vi "Create Digraph String.vi"(8 "Show Tag Labels?":bool, 9 "tag info":T3(array[cluster]), 10 "tables html":string[](array[string]), 11 "channel and node pairs":T1[](array[typedef])) -> (3 "digraph output":string)   [LabVIEW 2014, in "GraphViz Mapping Visualizer.lvlib"]
uses:
  GraphViz Mapping Visualizer.lvlib
  <vilib>/NI/Tag Bus/tag/Data Type.ctl
  Channel to Port Pair.ctl
  <vilib>/NI/Tag Bus/tag/tag descriptor.lvclass
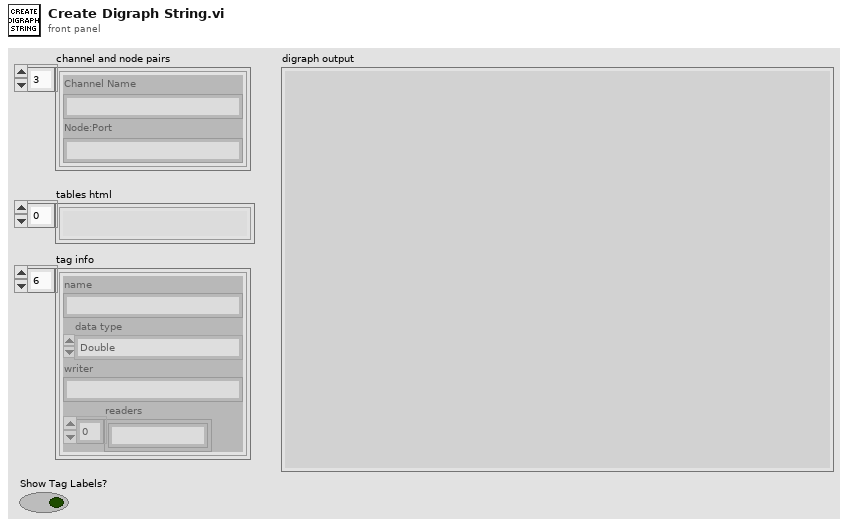
[diagram p1: front panel]
types:
  T1 = typedef "GraphViz Mapping Visualizer.lvlib/Channel to Port Pair.ctl" = cluster{"Channel Name":string, "Node:Port":string}
  T2 = typedef "tag bus.lvlib/tag descriptor.lvclass/Data Type.ctl" = enum16{"Double", "Single", "I64", "I32", "I16", "I8", "U64", "U32", "U16", "U8", "Boolean", "String", "Array of Double", "Array of Single", "Array of I64", "Array of I32", "Array of I16", "Array of I8", "Array of U64", "Array of U32", "Array of U16", "Array of U8", "Array of Boolean", "Array of String"}
  T3 = cluster{"name":string, "data type":T2, "writer":string, "readers":string[]}[]
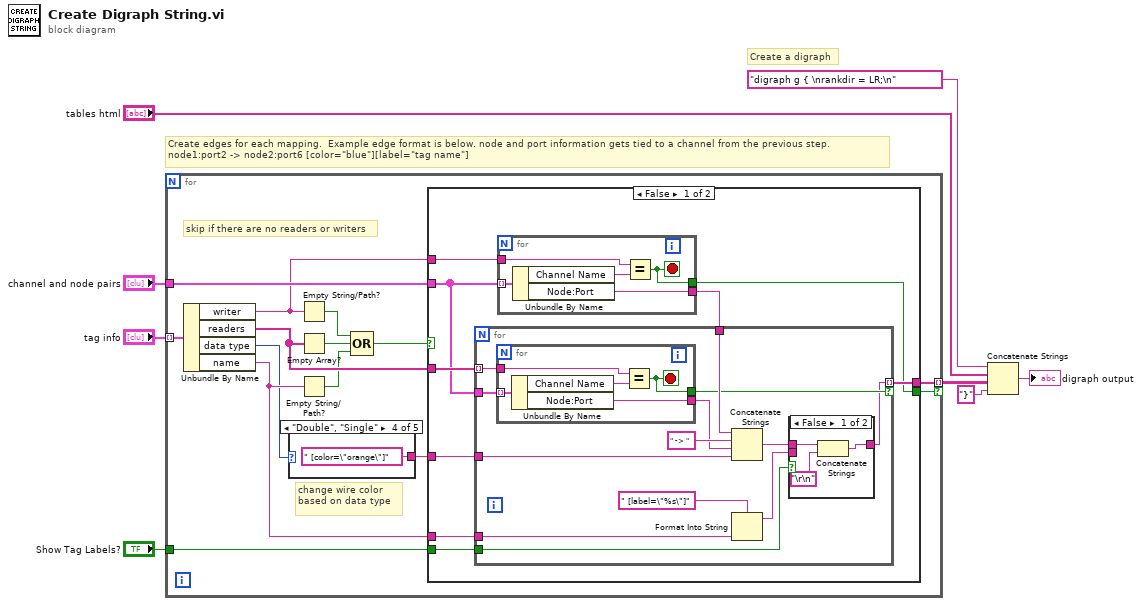
[diagram p0: block diagram]
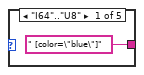
[diagram p2: hidden frame]
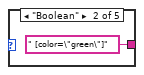
[diagram p3: hidden frame]
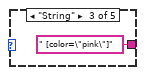
[diagram p4: hidden frame]
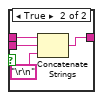
[diagram p6: hidden frame]
diagram:
  # "Create a digraph"
  # "Create edges for each mapping.  Example edge format is below. node and port information gets tied to a channel from the previous step.\nnode1:port2 -> node2:port6 [color=\"blue\"][label=\"tag name\"]"
  n1 = for {
    tunnel: "channel and node pairs" -> [w20]
    tunnel: [w19] -> w6 mode=indexing if=w18
    tunnel: "Show Tag Labels?" -> [w17]
    tunnel: "tag info" -> [w16] mode=indexing
    # "change wire color based on data type"
    # "skip if there are no readers or writers"
    n2 = Unbundle By Name(w16) -> ("writer"=w15:string, "readers"=w14:string[], "data type"=w9:T2, "name"=w12:string)
    n3 = case shown="\"Double\", \"Single\"" w9 {
      tunnel: [" [color=\"blue\"]" ("string") " [color=\"green\"]" ("string") " [color=\"pink\"]" ("string") " [color=\"orange\"]" ("string") _] -> w10
      frame "I64".."U8" {
      }
      frame "Boolean" {
      }
      frame "String" {
      }
      frame "Double", "Single" {
      }
      frame Default {
      }
    }
    n4 = Empty String/Path?(string/path=w15) -> (empty?=w13:bool)
    n5 = Empty Array?(array=w14) -> (empty?=w22:bool)
    n6 = Empty String/Path?(string/path=w12) -> (empty?=w11:bool)
    n7 = Compound Arithmetic op=OR(w13, w22, w11) -> (w21:bool)
    n8 = case shown="False" w21 {
      tunnel: w20 -> [w34 _]
      tunnel: w14 -> [w35 _]
      tunnel: w15 -> [w33 _]
      tunnel: w12 -> [w31 _]
      tunnel: [w30 _] -> w19
      tunnel: [w29 _] -> w18
      tunnel: w17 -> [w28 _]
      tunnel: w10 -> [w27 _]
      frame False {
        n9 = for {
          tunnel: w33 -> [w38]
          tunnel: w34 -> [w40] mode=indexing
          tunnel: [w37] -> w29
          tunnel: [w36] -> w32
          stop <- w37 stop-if-true
          n10 = Unbundle By Name(w40) -> ("Channel Name"=w39:string, "Node:Port"=w36:string)
          n11 = Equal?(x=w38, y=w39) -> (x = y?=w37:bool)
        }
        n12 = for {
          tunnel: w35 -> [w53] mode=indexing
          tunnel: w34 -> [w52]
          tunnel: w32 -> [w51]
          tunnel: w31 -> [w48]
          tunnel: [w42] -> w30 mode=indexing if=w46
          tunnel: w28 -> [w45]
          tunnel: w27 -> [w41]
          n13 = for {
            tunnel: w53 -> [w63]
            tunnel: w52 -> [w65] mode=indexing
            tunnel: [w62] -> w46
            tunnel: [w61] -> w47
            stop <- w62 stop-if-true
            n14 = Unbundle By Name(w65) -> ("Channel Name"=w64:string, "Node:Port"=w61:string)
            n15 = Equal?(x=w63, y=w64) -> (x = y?=w62:bool)
          }
          n16 = Concatenate Strings(w51, " -> " ("string"), w47, w41) -> (w43:string)
          n17 = Format Into String(format string=" [label=\"%s\"]" ("string"), w48) -> (resulting string=w44:string)  [unwired: 2 in, 1 out]
          n18 = case shown="False" w45 {
            tunnel: w44 -> [_ w59]
            tunnel: w43 -> [w56 w60]
            tunnel: [w54 w58] -> w42
            frame False {
              n19 = Concatenate Strings(w56, "\r\n") -> (w54:string)
            }
            frame True {
              n20 = Concatenate Strings(w60, w59, "\r\n") -> (w58:string)
            }
          }
        }
      }
      frame True {
      }
    }
  }
  n21 = Concatenate Strings("digraph g { \nrankdir = LR;\n", "tables html", w6, "}") -> (→"digraph output":string)
